vi "Intake Controller-test.vi"(8 "error in":errorcluster) -> ()   [LabVIEW 2017]
doc: "This VI executes continuously carrying out the current operation and responding to updates or new operation requests. It will often contain the timing or control code that is difficult to place directly in TeleOp. This VI generally opens all sensors and motors and isolates the rest of the robot code from knowing implementation details of how the operations are carried out."
uses:
  <vilib>/Rock Robotics/WPI/Framework/Completion Status.ctl
  Drive/Implementation/Drive Setpoints.ctl
  Drive/Implementation/Drive Operations.ctl
  <vilib>/Rock Robotics/WPI/SafetyOutput/WPI_SafetyOutputConfigMenu.ctl
  <vilib>/Rock Robotics/SystemInterfaces/DIO/FPGA_DIOChannel.ctl
  <vilib>/Rock Robotics/SystemInterfaces/DIO/FPGA_DIOPWMChannel.ctl
  <vilib>/Rock Robotics/WPI/Counter/WPI_CounterDigitalInputToDigitalSource.vi
  <vilib>/Rock Robotics/WPI/RobotDrive/WPI_RobotDriveOpen2MotorWithJaguar.vi
  <vilib>/Rock Robotics/WPI/ThirdParty/Sensors/navX/_Processing Loop/FRIC_navX_Internal_USB_ProcessingLoop.vi
panel:
  in  "Interactive Values":T1
  in  "Buttons":cluster{"Execute Cmd":bool, "Abort Cmd":bool}
  out "Command Timing":cluster{"Start Time (ms)":u32, "Iterations":i32}
  out "Status":T3
  out "Setpoints":T4(graph)
  out "Current\nCmd":string
  # "Tip: The graph shows the motor setpoints. It may also be helpful to observe inputs and sensor values.\nYou may also want to display tuning or debugging controls."
  # "Interactive Command: You may fill in the settings for a command\nand schedule it with the Execute button. You can observe and abort\nany command while fine tuning the code for the controller."
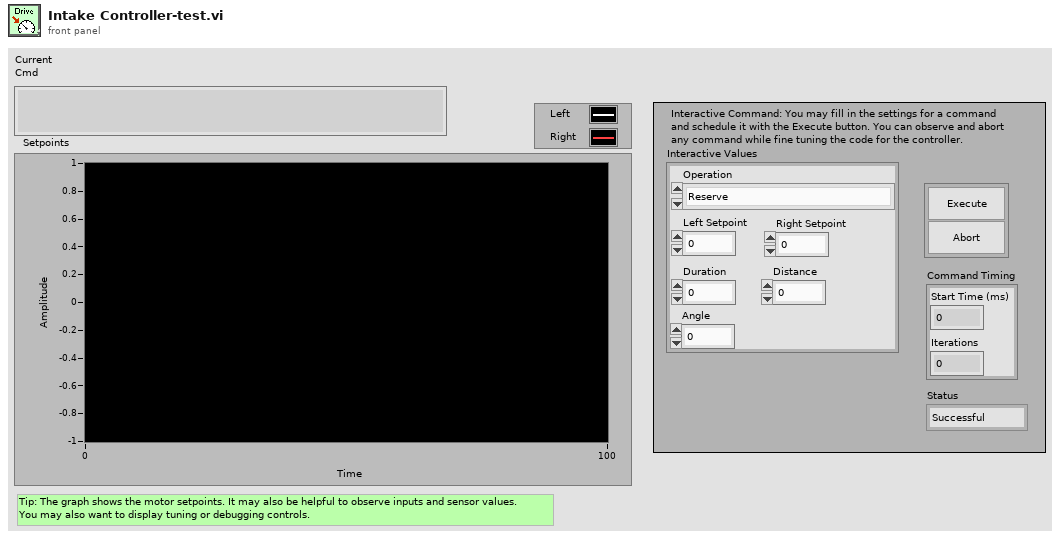
[diagram p1: front panel]
types:
  T1 = typedef "Drive Setpoints.ctl" = cluster{"Operation":T2, "Left Setpoint":dbl, "Right Setpoint":dbl, "Duration":dbl, "Distance":dbl, "Angle":dbl}
  T2 = typedef "Drive Operations.ctl" = enum16{"Reserve", "Read Current", "Immediate", "Drive for Angle", "Drive for Time", "Drive for Distance"}
  T3 = typedef "Completion Status.ctl" = enum16{"Successful", "Aborted", "Incomplete"}
  T4 = cluster{"Left Setpoint":dbl, "Right Setpoint":dbl}
  T5 = typedef "FPGA_DIOPWMChannel.ctl" = enum8{"PWM 0", "PWM 1", "PWM 2", "PWM 3", "PWM 4", "PWM 5", "PWM 6", "PWM 7", "PWM 8", "PWM 9", "PWM MXP 0", "PWM MXP 1", "PWM MXP 2", "PWM MXP 3", "PWM MXP 4", "PWM MXP 5", "PWM MXP 6", "PWM MXP 7", "PWM MXP 8", "PWM MXP 9", "Invalid"}
  T6 = typedef "FPGA_DIOChannel.ctl" = enum8{"DIO 0", "DIO 1", "DIO 2", "DIO 3", "DIO 4", "DIO 5", "DIO 6", "DIO 7", "DIO 8", "DIO 9", "DIO MXP 0", "DIO MXP 1", "DIO MXP 2", "DIO MXP 3", "DIO MXP 4", "DIO MXP 5", "DIO MXP 6", "DIO MXP 7", "DIO MXP 8", "DIO MXP 9", "DIO MXP 10", "DIO MXP 11", "DIO MXP 12", "DIO MXP 13", "DIO MXP 14", "DIO MXP 15", "SPI Port CS1", "SPI Port CS2", "SPI Port CS3", "SPI Port MISO", "SPI Port MOSI", "Invalid"}
  T7 = typedef "WPI_SafetyOutputConfigMenu.ctl" = enum16{"Enable", "Disable"}
  T8 = typedef "WPI_RobotDriveDevRef.ctl" = cluster{"DevStatus":errorcluster, "Motors[]":T9[], "Square Inputs":bool, "Max Output":dbl}
  T9 = typedef "WPI_MotorControlDeviceRef.ctl" = cluster{"DeviceStatus":errorcluster, "Type":T10, "PWM":cluster{"PWM Channel":T5, "DeadBand":T11}, "CAN":cluster{"Device Number":u8, "SetOutput VI Ref":variant, "GetOutput VI Ref":variant, "Enable VI Ref":variant, "Disable VI Ref":variant, "Data":variant}, "Invert":bool, "DIO PWM":cluster{"PWM \"Enable\" Channel":T5, "DIOChannel":T6, "PWM Rate":dbl}}
  T10 = typedef "WPI_MotorControlType.ctl" = enum16{"PWM", "CAN", "DIO PWM"}
  T11 = typedef "WPI_PWMDeadband.ctl" = cluster{"Name":string, "maxPositivePwm":i32, "minPositivePwm":i32, "centerPwm":i32, "maxNegativePwm":i32, "minNegativePwm":i32, "angularRange":u16}
  T12 = typedef "WPI_DigitalInputDevRef.ctl" = cluster{"DevStatus":errorcluster, "DIO Channel":T6}
  T13 = typedef "FPGA_CounterEncoderSourceConvertionLVSourceType.ctl" = cluster{"DevStatus":errorcluster, "AnalogTriggerMode?":bool, "DigitalMode":cluster{"DIO Channel":T14}, "AnalogTriggerMode":cluster{"AnalogTriggerIndex":T15, "OutputType":T16}}
  T14 = typedef "FPGA_DIODigitalSourceChannel.ctl" = enum8{"DIO 0", "DIO 1", "DIO 2", "DIO 3", "DIO 4", "DIO 5", "DIO 6", "DIO 7", "DIO 8", "DIO 9", "DIO MXP 0", "DIO MXP 1", "DIO MXP 2", "DIO MXP 3", "DIO MXP 4", "DIO MXP 5", "DIO MXP 6", "DIO MXP 7", "DIO MXP 8", "DIO MXP 9", "DIO MXP 10", "DIO MXP 11", "DIO MXP 12", "DIO MXP 13", "DIO MXP 14", "DIO MXP 15", "Disabled"}
  T15 = typedef "FPGA_AnalogTriggerIndex.ctl" = enum8{"Trig 0", "Trig 1", "Trig 2", "Trig 3", "Trig 4", "Trig 5", "Trig 6", "Trig 7", "Invalid"}
  T16 = typedef "FPGA_AnalogTriggerOutType.ctl" = enum16{"InWindow", "TriggerState", "Rising", "Falling"}
  T17 = typedef "WPI_EncoderDevRef.ctl" = cluster{"DevStatus":errorcluster, "EncoderIndex":T18, "CounterIndex":T19, "DistancePerCount":dbl, "Decoding Type":T20}
  T18 = typedef "FPGA_EncoderIdx.ctl" = enum8{"Enc 0", "Enc 1", "Enc 2", "Enc 3", "Enc 4", "Enc 5", "Enc 6", "Enc 7", "Invalid"}
  T19 = typedef "FPGA_CounterCtrSystemIndex.ctl" = enum8{"Ctr 0", "Ctr 1", "Ctr 2", "Ctr 3", "Ctr 4", "Ctr 5", "Ctr 6", "Ctr 7", "Invalid"}
  T20 = typedef "WPI_EncoderType.ctl" = enum16{"1x", "2x", "4x"}
  T21 = typedef "Command Status Info.ctl" = cluster{"Name":string, "Status":T3, "notifier out":T22}
  T22 = typedef "Completion Notifier.ctl" = refnum<notifier>
  T23 = cluster{"SubSystem Data":T1, cluster{"Start Time (ms)":u32, "Iterations":i32}, cluster{"Command Info":T21, "Description":string, "Default Command":T1, "queue out":refnum<queue>, "Subsystem Name":string}}
  T24 = cluster{"Yaw":dbl, "Roll":dbl, "Pitch":dbl, "Heading":dbl, "Fused Heading":dbl}
  T25 = cluster{"SubSystem Data":T1, cluster{"Start Time (ms)":u32, "Iterations":i32}, "Default Command Arguments":cluster{"Command Info":T21, "Description":string, "Default Command":T1, "queue out":refnum<queue>, "Subsystem Name":string}}
  T26 = cluster{"Don't move motors while reserved":dbl, "Don't move motors while reserved":dbl}
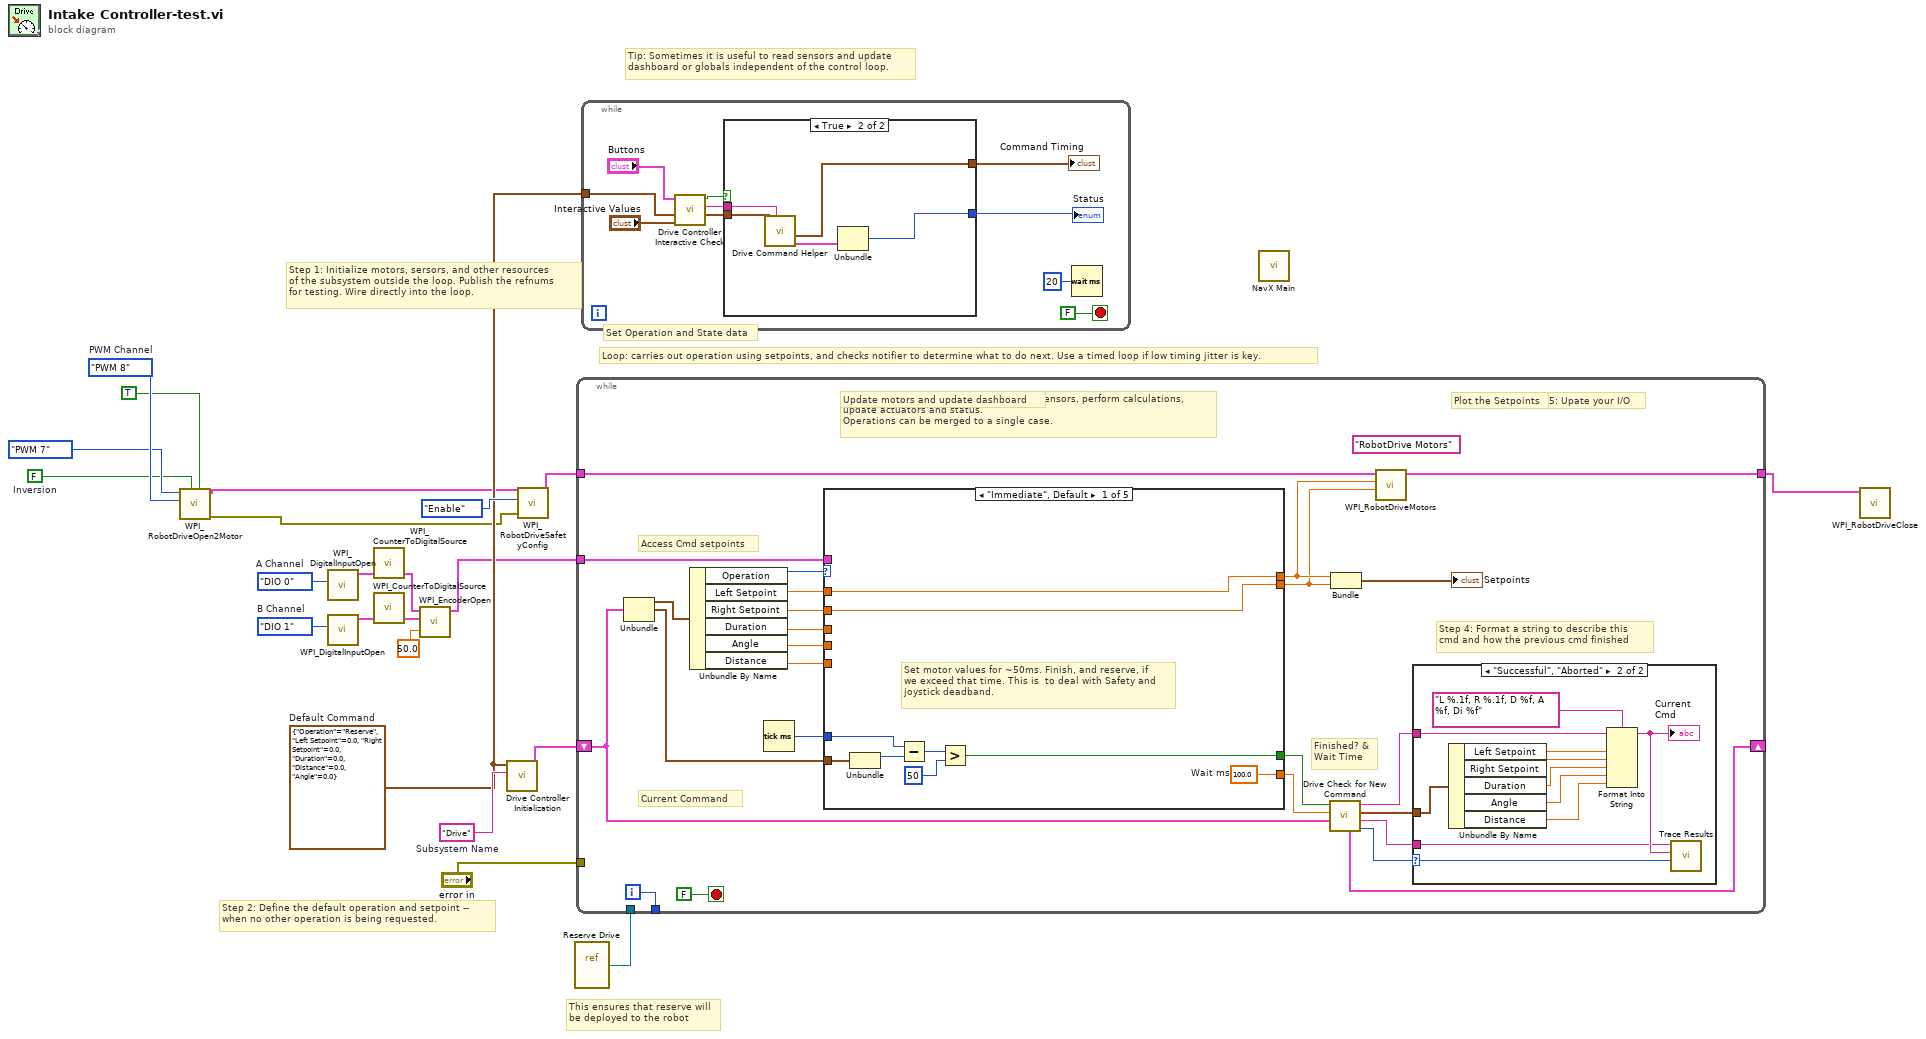
[diagram p0: block diagram]
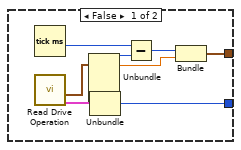
[diagram p2: hidden frame]
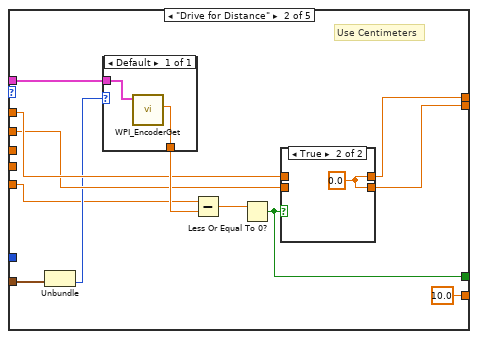
[diagram p4: hidden frame]
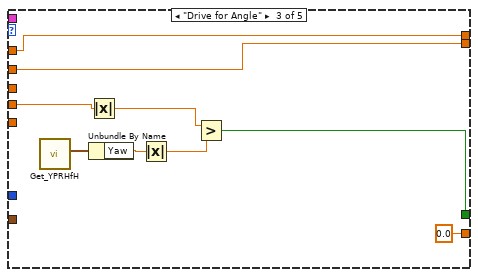
[diagram p6: hidden frame]
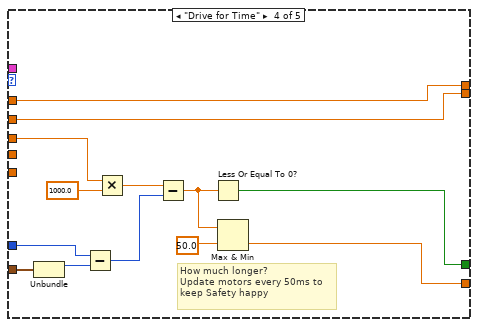
[diagram p7: hidden frame]
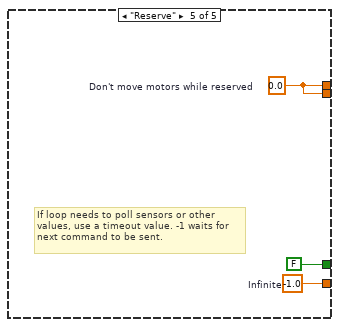
[diagram p8: hidden frame]
diagram:
  w2 = FALSE  # Inversion
  w4 = FPGA_DIOPWMChannel."PWM 8"  # PWM Channel
  w10 = FPGA_DIOChannel."DIO 1"  # B Channel
  w9 = FPGA_DIOChannel."DIO 0"  # A Channel
  w16 = T1 {"Operation"=enum."Reserve", "Left Setpoint"=0.0, "Right Setpoint"=0.0, "Duration"=0.0, "Distance"=0.0, "Angle"=0.0}  # Default Command
  w22 = "Drive"  # Subsystem Name
  # "Set Operation and State data"
  # "This ensures that reserve will\nbe deployed to the robot"
  # "Tip: Sometimes it is useful to read sensors and update\ndashboard or globals independent of the control loop."
  # "Step 2: Define the default operation and setpoint --\nwhen no other operation is being requested."
  # "Step 1: Initialize motors, sersors, and other resources\nof the subsystem outside the loop. Publish the refnums\nfor testing. Wire directly into the loop."
  # "Loop: carries out operation using setpoints, and checks notifier to determine what to do next. Use a timed loop if low timing jitter is key."
  n1 = call-poly <vilib>:"WPI_RobotDriveOpen2Motor.vi"("Right Motor Inverted"=TRUE ("Inversion"), "Left Motor Inverted"=w2, "Right Motor"=w4, "Left Motor"=FPGA_DIOPWMChannel."PWM 7" ("PWM Channel")) -> ("error out"=w5:errorcluster, "RobotDriveDevRef"=w6:T8)  [unwired: 6 in]
  n2 = call <vilib>:"WPI_DigitalInputOpen.vi"("DIO Channel"=w9) -> ("DigitalInputDevRef"=w13:T12)  [unwired: 1 in, 9 out]
  n3 = call <vilib>:"WPI_DigitalInputOpen.vi"("DIO Channel"=w10) -> ("DigitalInputDevRef"=w12:T12)  [unwired: 1 in, 9 out]
  n4 = call-poly <vilib>:"WPI_CounterToDigitalSource.vi"("DigitalInputDevRef"=w13) -> ("Digital Source"=w14:T13)  [unwired: 6 out]
  n5 = call-poly <vilib>:"WPI_CounterToDigitalSource.vi"("DigitalInputDevRef"=w12) -> ("Digital Source"=w11:T13)  [unwired: 6 out]
  n6 = call <vilib>:"WPI_EncoderOpen.vi"("DistancePerCount"=50.0, "BSource"=w11, "ASource"=w14) -> ("EncoderDevRef"=w7:T17)  [unwired: 5 in, 3 out]
  n7 = call "Drive Controller Initialization.vi"("Subsystem Name"=w22, "Default Command"=w16) -> ("Current Command"=w18:T23)  [unwired: 9 in]
  n8 = call <vilib>:"WPI_RobotDriveSafetyConfig.vi"("error in (no error)"=w5, "mode"=WPI_SafetyOutputConfigMenu."Enable", "RobotDriveDevRef"=w6) -> ("RobotDriveDevRef"=w20:T8)  [unwired: 7 in, 1 out]
  n9 = vi-ref "Reserve Drive.vi"() -> (w17:refnum<vi>)
  n10 = while {
    shift-right: [w34] -> _
    shift-left: w18 -> [w27]
    tunnel: [w46] -> _
    tunnel: w20 -> [w42]
    tunnel: "error in" -> [_]
    tunnel: w17 -> [_]
    tunnel: [w26] -> w15
    tunnel: w7 -> [w23]
    i -> [w46]
    stop <- FALSE stop-if-true
    (unwired) "RobotDrive Motors" ("Name")
    # "Step 5: Upate your I/O"
    # "Step 4: Format a string to describe this\ncmd and how the previous cmd finished"
    # "Current Command"
    # "Update motors and update dashboard"
    # "Plot the Setpoints"
    # "Access Cmd setpoints"
    # "Finished? &\nWait Time"
    # "Step 3: For a given operation, read from sensors, perform calculations,\nupdate actuators and status.\nOperations can be merged to a single case."
    n11 = Unbundle(w27) -> ("SubSystem Data"=w41:T1, w28:cluster{"Start Time (ms)":u32, "Iterations":i32})  [unwired: 1 out]
    n12 = Unbundle By Name(w41) -> ("Operation"=w40:T2, "Left Setpoint"=w39:dbl, "Right Setpoint"=w38:dbl, "Duration"=w37:dbl, "Angle"=w25:dbl, "Distance"=w24:dbl)
    n13 = Tick Count (ms)() -> (millisecond timer value=w36:u32)
    n14 = case shown="\"Immediate\", Default" w40 {
      tunnel: [w67 10.0 ("Infinite") 0.0 ("Infinite") w94 w109] -> w33
      tunnel: [w60 w72 w85 w101 FALSE ("ignore previous (F)")] -> w32
      tunnel: w28 -> [w59 w70 _ w103 _]
      tunnel: [w66 w75 w91 w100 w107] -> w44
      tunnel: [w65 w73 w92 w99 w107] -> w43
      tunnel: w39 -> [w66 w76 w91 w100 _]
      tunnel: w38 -> [w65 w74 w92 w99 _]
      tunnel: w37 -> [_ _ _ w98 _]
      tunnel: w36 -> [w61 _ _ w97 _]
      tunnel: w25 -> [_ _ w90 _ _]
      tunnel: w24 -> [_ w68 _ _ _]
      tunnel: w23 -> [_ w79 _ _ _]
      frame "Immediate", Default {
        w67 = 100.0  # Wait ms
        # "Set motor values for ~50ms. Finish, and reserve, if\nwe exceed that time. This is  to deal with Safety and\njoystick deadband."
        n15 = Unbundle(w59) -> ("Start Time (ms)"=w62:u32)  [unwired: 1 out]
        n16 = Subtract(x=w61, y=w62) -> (x-y=w63:u32)
        n17 = Greater?(x=w63, y=u8 50 ("Left Motor")) -> (0:w60:bool)
      }
      frame "Drive for Distance" {
        # "Use Centimeters"
        n18 = Unbundle(w70) -> ("Iterations"=w69:i32)  [unwired: 1 out]
        n19 = case shown="Default" w69 {
          tunnel: w79 -> [w84]
          tunnel: [w83] -> w78
          frame Default {
            n20 = call <vilib>:"WPI_EncoderGet.vi"("EncoderDevRef"=w84) -> ("Distance"=w83:dbl)  [unwired: 5 in, 5 out]
          }
        }
        n21 = Subtract(x=w68, y=w78) -> (x-y=w77:dbl)
        n22 = Less Or Equal To 0?(x=w77) -> (x <= 0?=w72:bool)
        n23 = case shown="True" w72 {
          tunnel: w76 -> [w81 _]
          tunnel: [w81 w82] -> w75
          tunnel: w74 -> [w80 _]
          tunnel: [w80 w82] -> w73
          frame False {
          }
          frame True {
            w82 = 0.0 ("Left Setpoint")
          }
        }
      }
      frame "Drive for Angle" {
        n24 = call <vilib>:"Get_YPRHfH.vi"() -> ("YRPHfH"=w89:T24)  [unwired: 11 in]
        n25 = Absolute Value(x=w90) -> (abs(x)=w86:dbl)
        n26 = Unbundle By Name(w89) -> ("Yaw"=w88:dbl)
        n27 = Absolute Value(x=w88) -> (abs(x)=w87:dbl)
        n28 = Greater?(x=w86, y=w87) -> (0:w85:bool)
      }
      frame "Drive for Time" {
        # "How much longer?\nUpdate motors every 50ms to\nkeep Safety happy"
        n29 = Unbundle(w103) -> ("Start Time (ms)"=w102:u32)  [unwired: 1 out]
        n30 = Subtract(x=w97, y=w102) -> (x-y=w106:u32)
        n31 = Multiply(x=w98, y=1000.0) -> (x*y=w105:dbl)
        n32 = Subtract(x=w105, y=w106) -> (x-y=w96:dbl)
        n33 = Less Or Equal To 0?(x=w96) -> (x <= 0?=w101:bool)
        n34 = Max & Min(x=w96, y=50.0) -> (min(x,y)=w94:dbl)  [unwired: 1 out]
      }
      frame "Reserve" {
        w107 = 0.0  # Don't move motors while reserved
        w109 = -1.0  # Infinite
        # "If loop needs to poll sensors or other\nvalues, use a timeout value. -1 waits for\nnext command to be sent."
      }
    }
    n35 = call "Drive Check for New Command.vi"("input cluster"=w27, "Wait time (ms)"=w33, "Finished?"=w32) -> ("Completion"=w35:T3, "Subsystem Name"=w29:string, "Current Command"=w30:T1, "Initial Trace String"=w31:string, "Next Command"=w34:T25)  [unwired: 4 in]
    n36 = Bundle("Don't move motors while reserved"=w44, "Don't move motors while reserved"=w43) -> (→"Setpoints":T26)  [unwired: 1 in]
    n37 = call <vilib>:"WPI_RobotDriveMotors.vi"("RightSpeed"=w43, "LeftSpeed"=w44, "RobotDriveDevRef"=w42) -> ("RobotDriveDevRef"=w26:T8)  [unwired: 1 in, 7 out]
    n38 = case shown="\"Successful\", \"Aborted\"" w35 {
      selector: w35 -> [_ w58]
      tunnel: w31 -> [_ w53]
      tunnel: w30 -> [_ w54]
      tunnel: w29 -> [_ w50]
      frame "Incomplete", Default {
        # "Continuing current command"
      }
      frame "Successful", "Aborted" {
        # "Report and setup for next command"
        n39 = Unbundle By Name(w54) -> ("Left Setpoint"=w56:dbl, "Right Setpoint"=w57:dbl, "Duration"=w51:dbl, "Angle"=w49:dbl, "Distance"=w48:dbl)
        n40 = Format Into String(format string="L %.1f, R %.1f, D %f, A %f, Di %f", initial string=w53, w56, w57, w51, w49, w48) -> (resulting string=w52:string)  [unwired: 1 in, 1 out]
        "Current\nCmd" <- w52
        n41 = call <vilib>:"Trace Results.vi"("Status of previous command"=w58, "Description"=w52, "Subsystem"=w50) -> ()  [unwired: 9 in]
      }
    }
  }
  n42 = while {
    tunnel: w16 -> [w111]
    stop <- FALSE stop-if-true
    n43 = call "Drive Controller Interactive Check.vi"("Interactive Command In"="Interactive Values", "Default Command"=w111, "Buttons"="Buttons") -> ("Interactive Command Out"=w113:T1, "Trace String"=w114:string, "Schedule"=w115:bool)  [unwired: 6 in]
    n44 = case shown="True" w115 {
      tunnel: [w124 w132] -> w116
      tunnel: [w123 w128] -> w117
      tunnel: w114 -> [_ w130]
      tunnel: w113 -> [_ w129]
      frame False {
        n45 = Tick Count (ms)() -> (millisecond timer value=w127:u32)
        n46 = call "Read Drive Operation.vi"() -> ("Command Info"=w121:T21, "SubSystem Data"=w120:T1)  [unwired: 9 in, 1 out]
        n47 = Unbundle(w120) -> ("Operation"=w125:T2, "Left Setpoint"=w122:dbl)  [unwired: 4 out]
        n48 = Unbundle(w121) -> ("Status"=w124:T3)  [unwired: 2 out]
        n49 = Subtract(x=w127, y=w125) -> (x-y=w126:u32)
        n50 = Bundle(w126, "Left Setpoint"=w122) -> (w123:cluster{u32, "Left Setpoint":dbl})  [unwired: 1 in]
      }
      frame True {
        n51 = call "Drive Command Helper.vi"("Description"=w130, "SubSystem Data"=w129) -> ("Command Info Out"=w131:T21, "Command Timing"=w128:cluster{"Start Time (ms)":u32, "Iterations":i32})  [unwired: 7 in, 1 out]
        n52 = Unbundle(w131) -> ("Status"=w132:T3)  [unwired: 2 out]
      }
    }
    "Status" <- w116
    "Command Timing" <- w117
    n53 = Wait (ms)(milliseconds to wait=u32 20) -> ()  [unwired: 1 out]
  }
  n54 = call-poly <vilib>:"NavX Main.vi"() -> ()  [unwired: 12 in]
  n55 = call <vilib>:"WPI_RobotDriveClose.vi"("RobotDriveDevRef"=w15) -> ()  [unwired: 10 in, 1 out]
